vi "Multi_Point_TraverseControl.vi"(0 "Mode":T2=enum."Read traverse position", 1 "Route Checking?":bool, 3 "Traverse Name":string, 5 "RollPitchYaw":dbl[](array[numeric]) caption="Model       Roll      Pitch       Yaw (deg)" format="%#.2f", 9 "Points to plot":dbl[][](array[numeric]) format="%.2f", 11 "Work in Tunnel Coordinates?":T1, 13 "Speed Factor":dbl=1.0 min=0.1 max=5.0 format="%.2f", 14 "Backlash Compensation?":bool=TRUE) -> (4 "Position Output XYZ":dbl[](array[numeric]) format="%.2f", 15 "Error String":string)   [LabVIEW 2013]
uses:
  Anemometry/Anemometry Sub Vis/Gen Trav/Trav_mode.ctl
  Anemometry/Anemometry Sub Vis/Controls/Tunnel_Coordinates.ctl
  ~subVIs/GenericDriveCommand.ctl
  ADAM Client/Sub VIs/ADAM Controls/Update_scan_value.ctl
  Anemometry/Anemometry Sub Vis/Globals/Trav_pos_global.vi
  Anemometry/Anemometry Sub Vis/Globals/Preference_global.vi
  ~subVIs/DriveConfigGlobal.vi
  Anemometry/Anemometry Sub Vis/Gen Trav/Route mapping/Route_mapping_global.vi
panel:
  out "Server copy Location":path
  out "Log File":path
  out "Achieved Pos In Eng units of all channels":dbl[](array[numeric]) format="%.2f"
  out "Pulses Positon all channels":dbl[](array[numeric])
  out "Counters Reset?":bool
  # "X                Y                   Z"
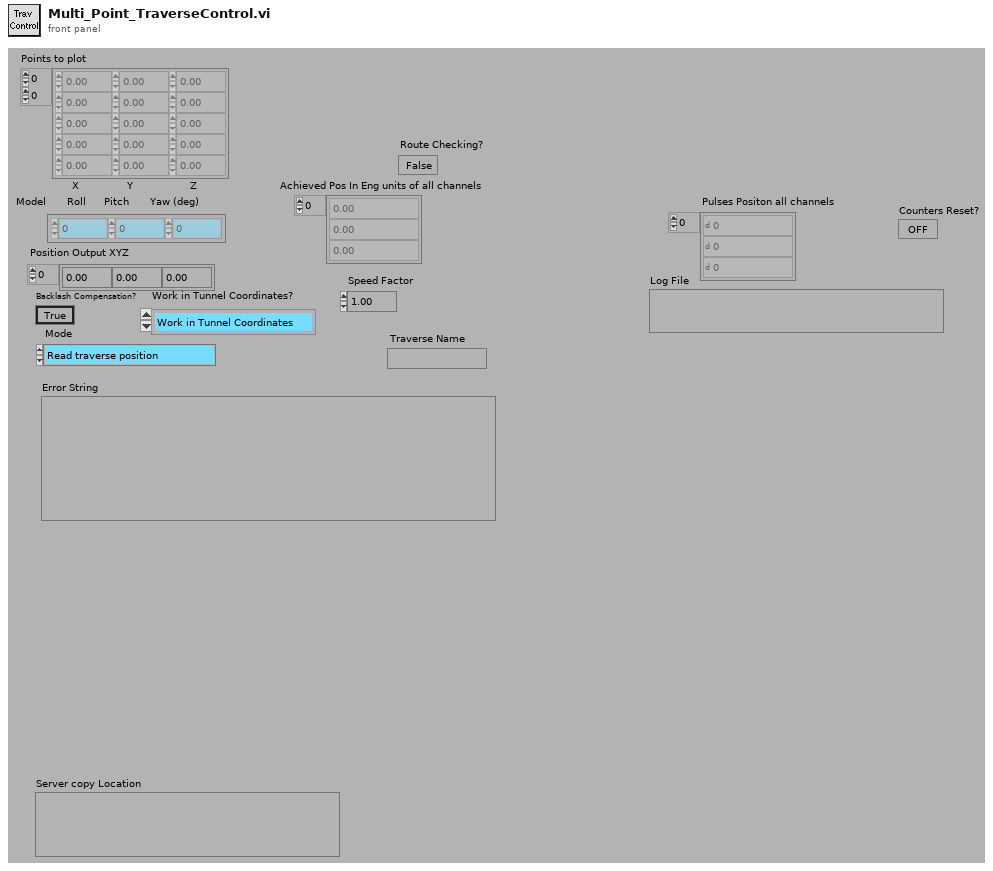
[diagram p1: front panel]
types:
  T1 = typedef "Tunnel_Coordinates.ctl" = enum16{"Work in Tunnel Coordinates", "Work in Model Coordinates"}
  T2 = typedef "Trav_mode.ctl" = enum16{"Move traverse", "Read traverse position", "Teach Position"}
  T3 = typedef "GenericDriveCommand.ctl" = string
  T4 = enum16{"To Traverse Coordinates", "To User Coordinates"}
  T5 = typedef "Update_scan_value.ctl" = cluster{"Channel Name":string, "New Value":dbl}
  T6 = typedef "AxisConfigCluster.ctl" = cluster{"Channel Properties":T7, "Static Drive Configuration":T8}
  T7 = typedef "DriveProperties.ctl" = cluster{"Channel Name":string, "Vel. Default":dbl, "Acc. Default":dbl, "Vel. Max":dbl, "Vel. Min":dbl, "Acc. Max":dbl, "Acc. Min":dbl, "Pulses/unit":dbl, "Address":u8, "Pulse Offset":i32, "Pos Tolerance":dbl, "Pulses/rev":dbl, "Backlash/Eng units":dbl, "Current Pos":dbl, "Ch Status":enum16{"Active", "Offline", "Simulate"}, "Port Name":string, "Axis Transform mode":string, "Metadata Ch Name":string, "Type":string}
  T8 = typedef "DriveStaticConfig.ctl" = cluster{"Correction Gain % (CG)":u16, "Dead Band (DB)":i32, "Dead Band Window (DW)":i32, "Encoder Resolution (ER)":i32, "Step Mode  (FSB)":u16, "Position Maintenance (FSC)":u16, "Stop on Stall (FSD)":u16, "Activate OP1 on stall (FSE)":u16, "Stop on Trigger 3 (FSF)":u16, "OP2 in Deadband (FSG)":u16, "Stall Detect (FSH)":u16, "Limit Disable (LD)":u16, "Motor Resolution (MR)":enum16{"200", "400", "1000", "2000", "4000", "5000", "10000", "12800", "18000", "20000", "21600", "25000", "25400", "25600", "36000", "50000", "278528", "425984", "507904", "614400", "655360", "819200", "1024000"}, "Limit Switch Sense (OSA)":u16, "Home Position (OSB)":u16, "Home Switch Sense (OSC)":u16, "Encoder Z for Home (OSD)":u16, "Reference edge of Home (OSH)":u16, "RS232 Echo Control (SSA)":u16, "Buffer at Limit (SSG)":u16, "Buffer at Stop (SSH)":u16, "Indexer Mode  (FSA)":u16, "Type":string, "ConfigString":string, "De Power Motor":enum16{"TRUE", "FALSE"}}
  T9 = typedef "Box_size.ctl" = cluster{"Max":dbl, "Min":dbl}[]
  T10 = typedef "Exclude_cluster.ctl" = cluster{"Sizes":T9, "Name":string, "Exclude Type":T11}
  T11 = typedef "Exclusion_type.ctl" = enum16{"Exclude completely", "Allow only vertical moves"}
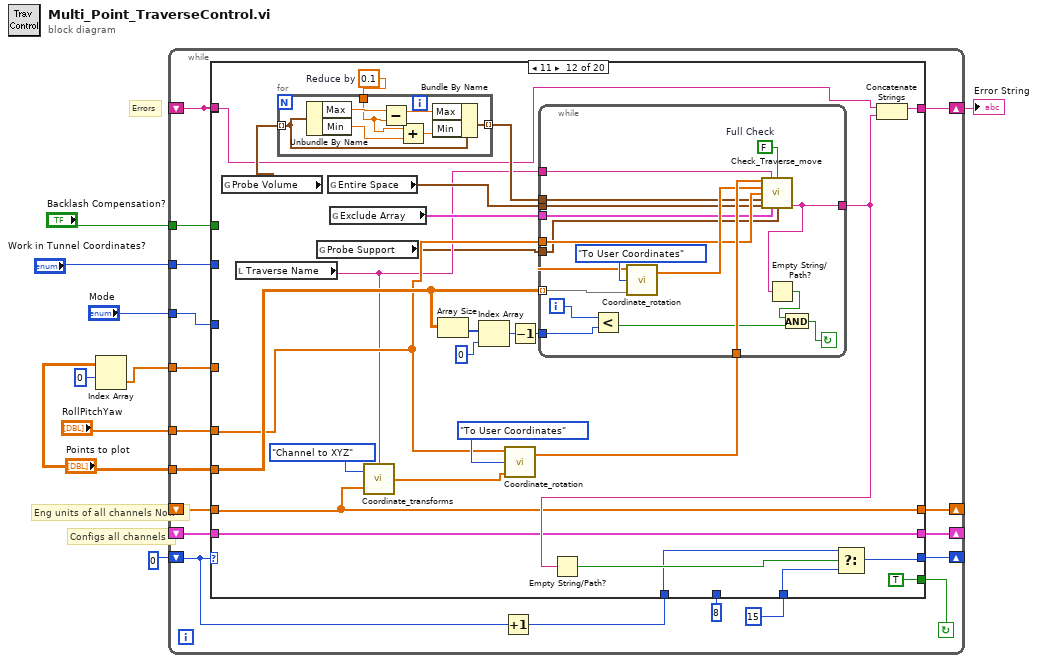
[diagram p0: block diagram]
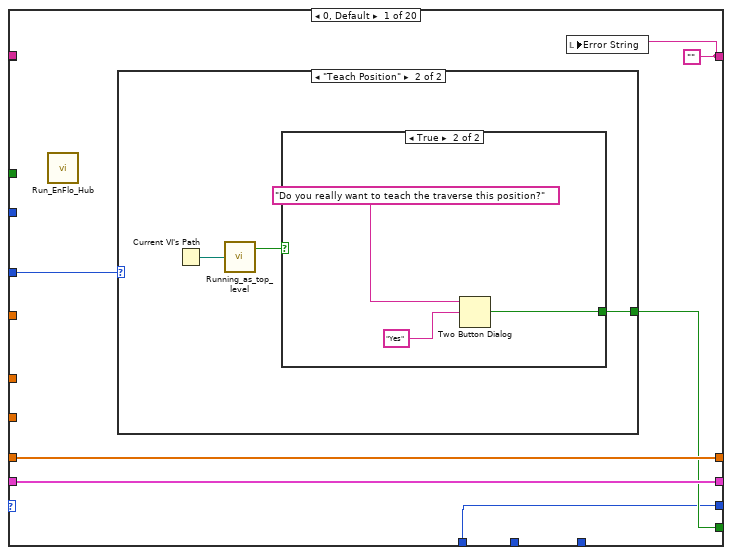
[diagram p2: hidden frame]
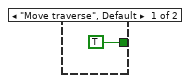
[diagram p3: hidden frame]
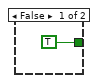
[diagram p4: hidden frame]
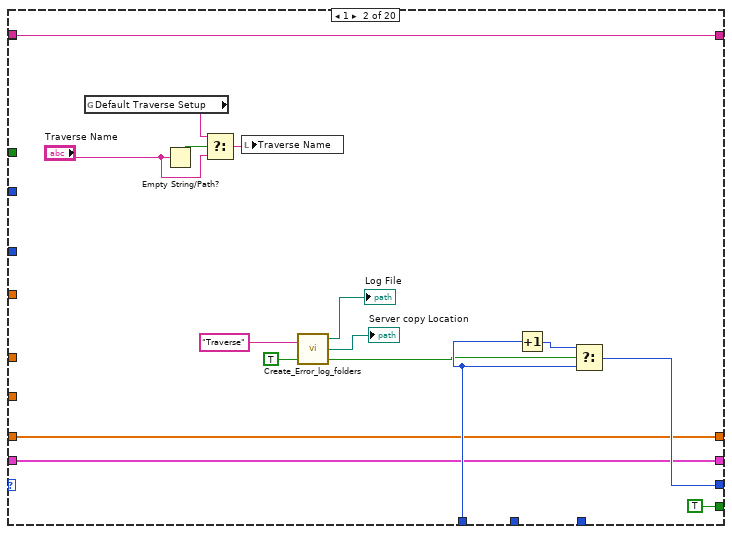
[diagram p5: hidden frame]
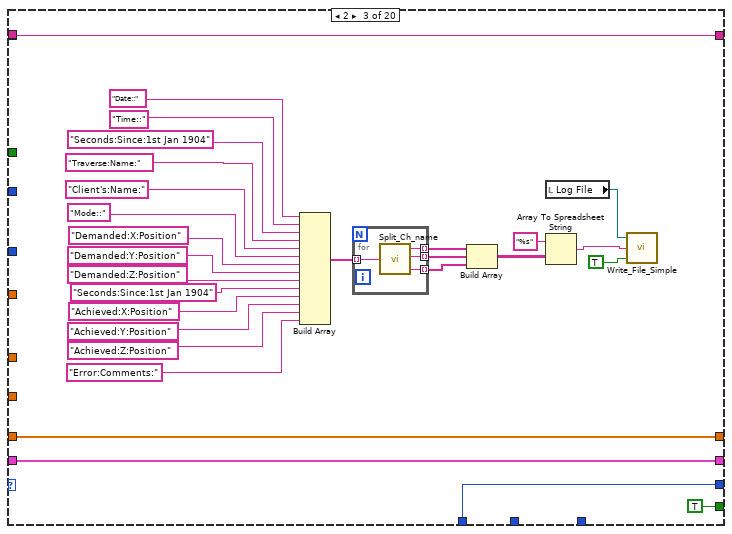
[diagram p6: hidden frame]
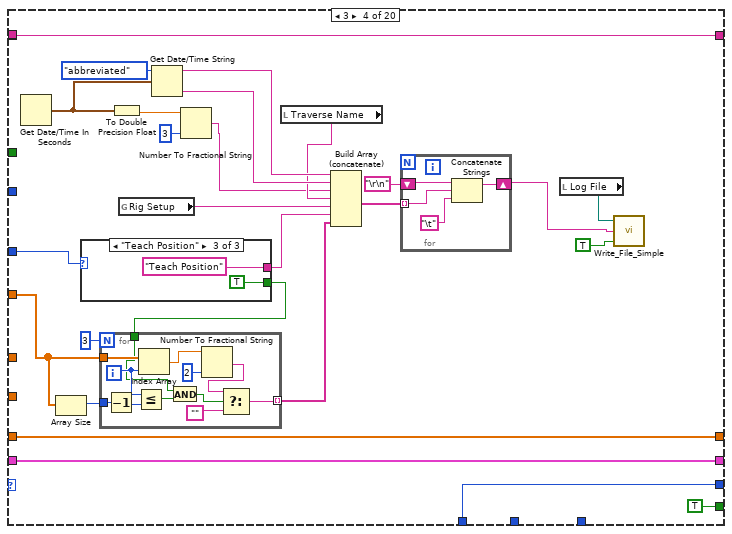
[diagram p7: hidden frame]
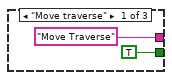
[diagram p8: hidden frame]
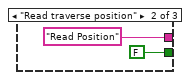
[diagram p9: hidden frame]
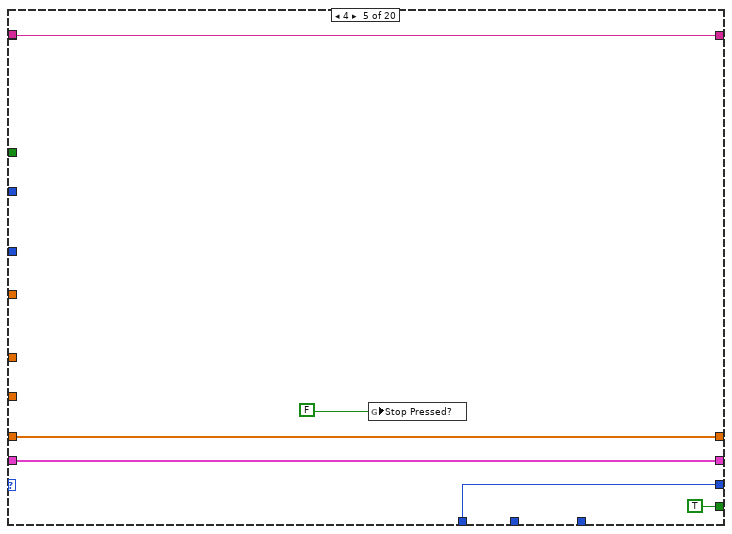
[diagram p10: hidden frame]
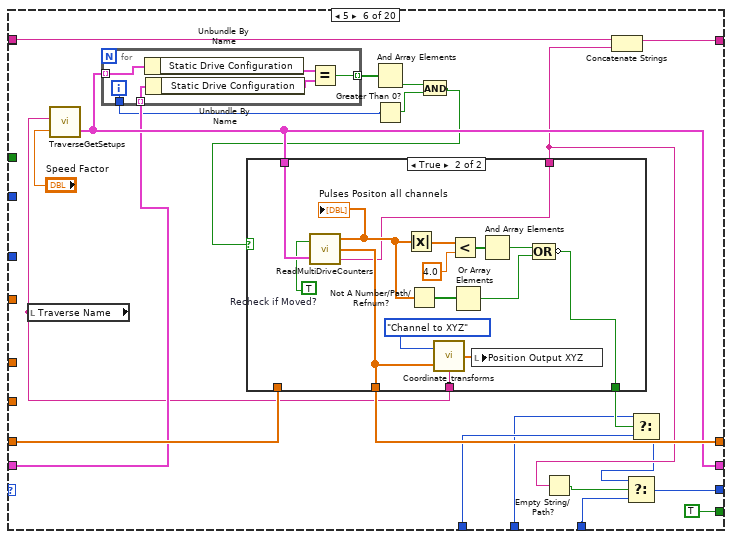
[diagram p11: hidden frame]
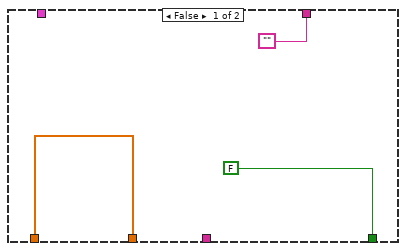
[diagram p12: hidden frame]
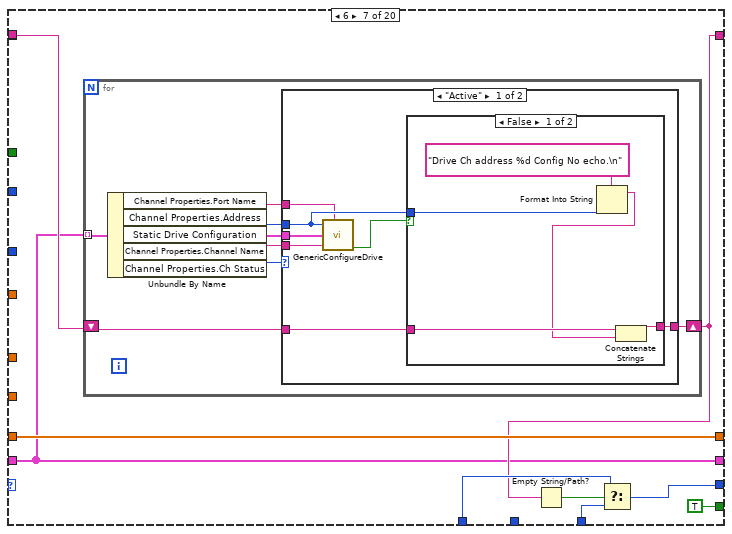
[diagram p13: hidden frame]
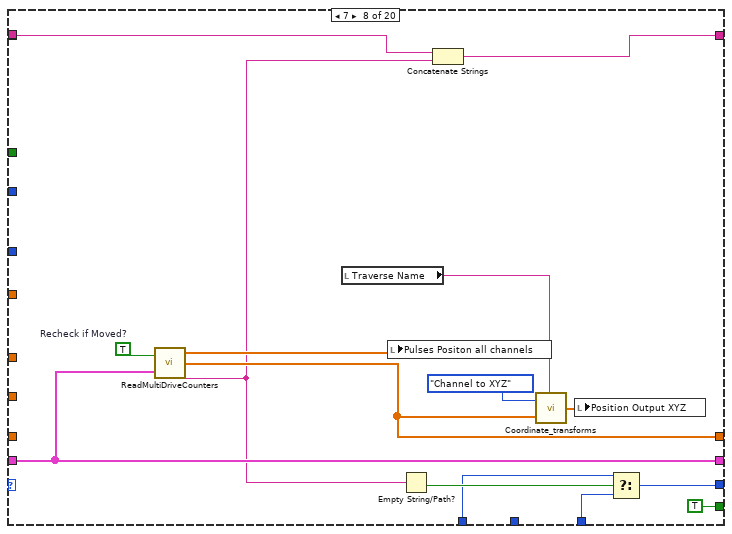
[diagram p16: hidden frame]
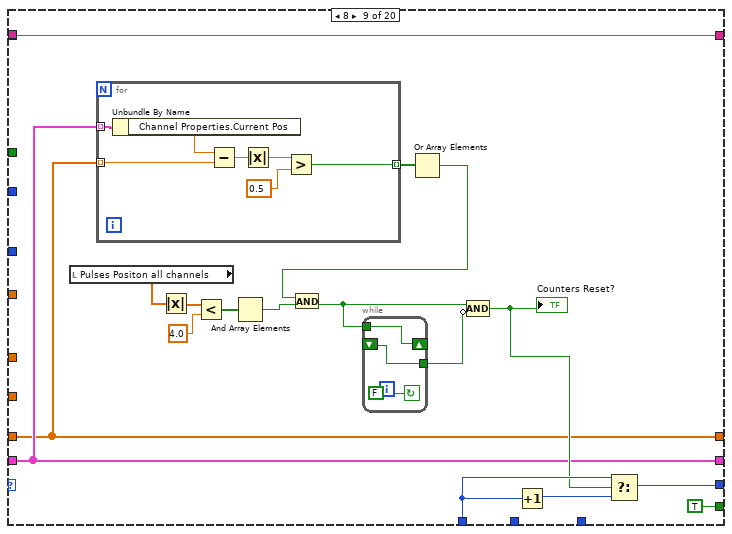
[diagram p17: hidden frame]
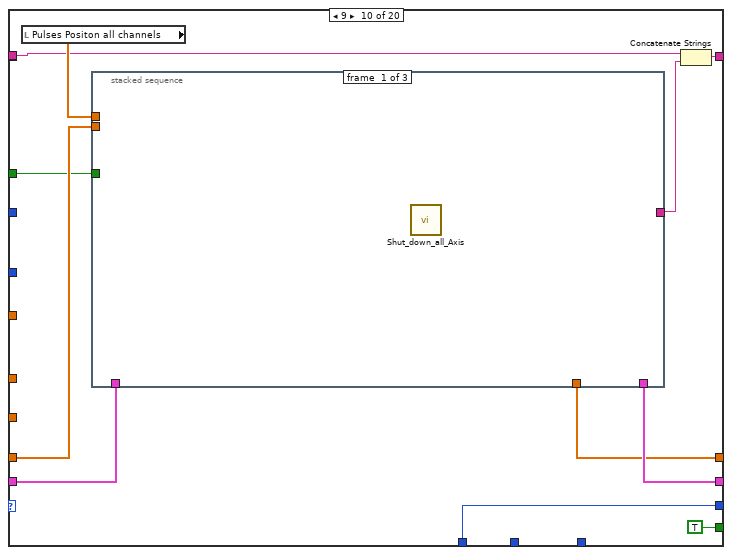
[diagram p18: hidden frame]
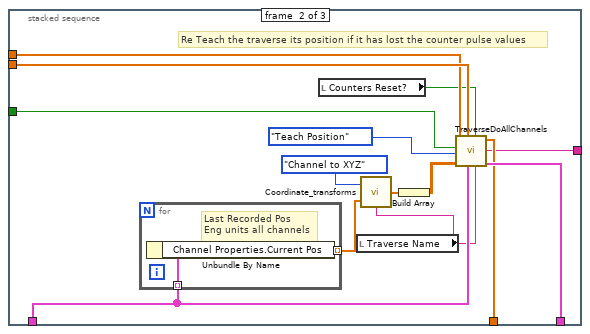
[diagram p19: hidden frame]
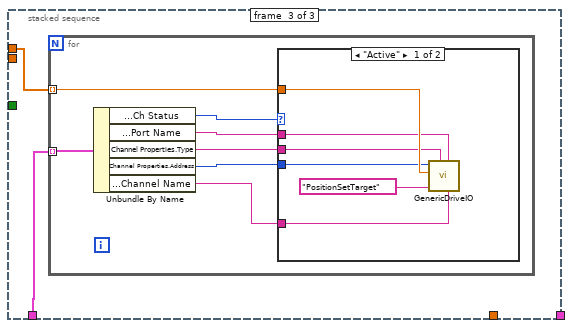
[diagram p20: hidden frame]
diagram:
  # "Errors"
  # "Eng units of all channels Now"
  # "Configs all channels"
  n1 = Index Array(array="Points to plot", index (row)=0) -> (element=w4:dbl[])  [unwired: 1 in]
  n2 = while {
    tunnel: "Backlash Compensation?" -> [w13]
    tunnel: w4 -> [w17]
    shift-left: _ -> [w14]
    shift-right: [w18] -> w7
    shift-left: _ -> [w19]
    shift-right: [w20] -> _
    shift-left: _ -> [w21]
    shift-right: [w22] -> _
    shift-left: 0 -> [w25]
    shift-right: [w23] -> _
    tunnel: "Mode" -> [w27]
    tunnel: "RollPitchYaw" -> [w12]
    tunnel: "Work in Tunnel Coordinates?" -> [w11]
    tunnel: "Points to plot" -> [w10]
    stop <- w26 continue-if-true
    n3 = Increment(x=w25) -> (x+1=w24:i32)
    n4 = case shown="11" w25 {
      tunnel: w27 -> [w33 _ _ w108 _ _ _ _ _ _ w310 _ w375 w405 _ _ _ w481 _ w537]
      tunnel: [w30 TRUE ("T button?") TRUE ("T button?") TRUE ("T button?") TRUE TRUE ("T button?") TRUE ("T button?") TRUE ("T button?") TRUE TRUE TRUE ("T button?") TRUE ("T button?") TRUE TRUE TRUE ("T button?") TRUE ("T button?") TRUE ("T button?") w483 TRUE FALSE] -> w26
      tunnel: w24 -> [w29 w56 w65 w113 w138 w162 w195 w223 w248 w264 w309 w325 w382 w407 w433 w447 w476 w480 w515 w544]
      tunnel: [w29 w54 w65 w113 w138 w145 w194 w221 w246 w264 w308 w323 w382 w406 w433 w445 w476 w479 w515 w544] -> w23
      tunnel: [w31 w51 w67 w115 w140 w160 w190 w235 w242 w273 w306 w329 w376 w404 w435 w459 w478 w486 w513 w542] -> w22
      tunnel: w21 -> [w31 w51 w67 w115 w140 w159 w190 w235 w242 w272 w306 w329 w389 w404 w435 w459 w478 w486 w513 w542]
      tunnel: [w32 w52 w66 w114 w141 w165 w198 w230 w241 w269 w305 w328 w383 w410 w434 w458 w477 w487 w516 w545] -> w20
      tunnel: w19 -> [w32 w52 w66 w114 w141 w164 w198 _ w241 w270 w305 w328 w378 w410 w434 w458 w477 w487 w516 w545]
      tunnel: [w28 w50 w63 w105 w142 w150 w191 w226 w245 w266 w311 w326 w385 w408 w431 w449 w474 w482 w509 w538] -> w18
      tunnel: w14 -> [_ w50 w63 w105 w142 w151 w192 w227 w245 w268 w311 w327 w386 w408 w431 w449 w474 w485 w511 w540]
      tunnel: w17 -> [_ _ _ w102 _ _ _ _ _ _ _ _ _ _ _ _ _ _ w507 _]
      tunnel: 15 ("f") -> [_ _ _ _ _ w146 w193 w222 _ _ _ w324 _ _ _ _ _ _ _ _]
      tunnel: 8 ("t") -> [_ _ _ _ _ w161 _ _ _ _ _ _ _ _ _ _ _ _ _ _]
      tunnel: w14 -> [_ _ _ _ _ _ _ _ _ _ _ _ _ _ _ _ _ _ _ _]
      tunnel: w13 -> [_ _ _ _ _ _ _ _ _ w263 _ _ w377 _ _ _ _ _ _ _]
      tunnel: w12 -> [_ _ _ _ _ _ _ _ _ _ _ w330 w373 _ _ _ _ _ w508 w535]
      tunnel: w11 -> [_ _ _ _ _ _ _ _ _ _ _ _ w372 _ _ _ _ _ w505 w533]
      tunnel: w10 -> [_ _ _ _ _ _ _ _ _ _ _ w331 w374 _ _ _ _ _ _ _]
      frame 0, Default {
        w28 = ""
        n5 = call "Run_EnFlo_Hub.vi"() -> ()  [unwired: 8 out]
        n6 = case shown="\"Teach Position\"" w33 {
          tunnel: [TRUE ("T button?") w35] -> w30
          frame "Move traverse", Default {
          }
          frame "Teach Position" {
            n7 = Current VI's Path() -> (path=w37:path)
            n8 = call "Running_as_top_level.vi"("Vi path name"=w37) -> ("Top Level"=w36:bool)  [unwired: 1 out]
            n9 = case shown="True" w36 {
              tunnel: [TRUE ("T button?") w39] -> w35
              frame False {
              }
              frame True {
                n10 = Two Button Dialog(message="Do you really want to teach the traverse this position?", 2:"Yes" ("T button name (\"OK\")")) -> (T button?=w39:bool)  [unwired: 1 out]
              }
            }
          }
        }
        n11 = local write "Error String"(w28) -> ()
      }
      frame 1 {
        n12 = global read "Trav_pos_global.vi" "Default Traverse Setup"() -> (w47:string)
        n13 = Empty String/Path?(string/path="Traverse Name") -> (empty?=w45:bool)
        n14 = Select(t=w47, s=w45, f="Traverse Name") -> (s? t:f=w44:string)
        n15 = local write "Traverse Name"(w44) -> ()
        n16 = call "Create_Error_log_folders.vi"("Per Day Log File?"=TRUE, "Log Filename"="Traverse" ("Input Element")) -> ("exists?"=w48:bool, "Server copy Location"=→"Server copy Location":path, "Local Log File"=→"Log File":path)  [unwired: 1 in]
        n17 = Increment(x=w56) -> (x+1=w55:i32)
        n18 = Select(t=w55, s=w48, f=w56) -> (s? t:f=w54:i32)
      }
      frame 2 {
        n19 = Build Array("Date::", "Time::", "Seconds:Since:1st Jan 1904", "Traverse:Name:", "Client's:Name:", "Mode::", "Demanded:X:Position", "Demanded:Y:Position", "Demanded:Z:Position", "Seconds:Since:1st Jan 1904", "Achieved:X:Position", "Achieved:Y:Position", "Achieved:Z:Position", "Error:Comments:") -> (w70:string[])
        n20 = for {
          tunnel: w70 -> [w89] mode=indexing
          tunnel: [w88] -> w71 mode=indexing
          tunnel: [w87] -> w72 mode=indexing
          tunnel: [w86] -> w73 mode=indexing
          n21 = call "Split_Ch_name.vi"("Ch name"=w89) -> ("Top level"=w88:string, "Middle"=w87:string, "Low level"=w86:string)
        }
        n22 = Build Array(w71, w72, w73) -> (w68:string[][])
        n23 = local read "Log File"() -> (w59:path)
        n24 = Array To Spreadsheet String(array=w68, 3:"%s" ("format string")) -> (spreadsheet string=w60:string)  [unwired: 1 out]
        n25 = call "Write_File_Simple.vi"("append to file? (new file:F)"=TRUE, "character string"=w60, "file path"=w59) -> ()  [unwired: 2 out]
      }
      frame 3 {
        n26 = Get Date/Time In Seconds() -> (seconds since 1Jan1904=w94:timestamp)
        n27 = Array Size(array=w102) -> (size(s)=w103:i32)
        n28 = case shown="\"Teach Position\"" w108 {
          tunnel: ["Move Traverse" "Read Position" "Teach Position"] -> w109
          tunnel: [TRUE FALSE TRUE] -> w99
          frame "Move traverse" {
          }
          frame "Read traverse position" {
          }
          frame "Teach Position" {
          }
        }
        n29 = for {
          N: 3 -> [_]
          tunnel: w102 -> [w127]
          tunnel: w103 -> [w124]
          tunnel: [w120] -> w100 mode=indexing
          tunnel: w99 -> [w116]
          i -> [w122]
          n30 = Decrement(x=w124) -> (x-1=w123:i32)
          n31 = Less Or Equal?(x=w122, y=w123) -> (x <= y?=w118:bool)
          n32 = Index Array(array=w127, index=w122) -> (element=w126:dbl)
          n33 = And(x=w116, y=w118) -> (x .and. y?=w117:bool)
          n34 = Number To Fractional String(number=w126, precision (6)=i16 2) -> (F-format string=w121:string)  [unwired: 2 out]
          n35 = Select(t=w121, s=w117, f="") -> (s? t:f=w120:string)
        }
        n36 = To Double Precision Float(number=w94) -> (double precision float=w93:dbl)
        n37 = global read "Preference_global.vi" "Rig Setup"() -> (w90:string)
        n38 = Get Date/Time String(date format (0)=enum16{"short", "long", "abbreviated"}."abbreviated", seconds (now)=w94) -> (date string=w111:string, time string=w110:string)  [unwired: 1 out]
        n39 = Number To Fractional String(number=w93, precision (6)=i16 3) -> (F-format string=w91:string)  [unwired: 2 out]
        n40 = local read "Traverse Name"() -> (w95:string)
        n41 = Build Array (concatenate)(w111, w110, w91, w95, w90, w109, w100) -> (w106:string[])
        n42 = for {
          shift-right: [w130] -> w96
          shift-left: "\r\n" -> [w131]
          tunnel: w106 -> [w129] mode=indexing
          n43 = Concatenate Strings(w131, w129, "\t") -> (w130:string)
        }
        n44 = local read "Log File"() -> (w97:path)
        n45 = call "Write_File_Simple.vi"("append to file? (new file:F)"=TRUE, "character string"=w96, "file path"=w97) -> ()  [unwired: 2 out]
      }
      frame 4 {
        n46 = global write "DriveConfigGlobal.vi" "Stop Pressed?"(FALSE) -> ()
      }
      frame 5 {
        n47 = local read "Traverse Name"() -> (w153:string)
        n48 = call "TraverseGetSetups.vi"("Speed Factor"="Speed Factor", "Traverse Name"=w153) -> ("Matched Configurations"=w160:T6[])  [unwired: 1 out]
        n49 = for {
          tunnel: w160 -> [w171] mode=indexing
          tunnel: w159 -> [w170] mode=indexing
          tunnel: [w167] -> w158 mode=indexing
          tunnel: [w166] -> w157
          i -> [w166]
          n50 = Unbundle By Name(w171) -> ("Static Drive Configuration"=w169:T8)
          n51 = Unbundle By Name(w170) -> ("Static Drive Configuration"=w168:T8)
          n52 = Equal?(x=w169, y=w168) -> (x = y?=w167:bool)
        }
        n53 = And Array Elements(Boolean array=w158) -> (logical AND=w155:bool)
        n54 = Greater Than 0?(x=w157) -> (x > 0?=w156:bool)
        n55 = And(x=w155, y=w156) -> (x .and. y?=w154:bool)
        n56 = case shown="True" w154 {
          tunnel: w160 -> [_ w189]
          tunnel: [w174 w179] -> w165
          tunnel: w164 -> [w174 _]
          tunnel: [FALSE w181] -> w163
          tunnel: w153 -> [_ w177]
          tunnel: ["" w175] -> w149
          frame False {
          }
          frame True {
            w176 = TRUE  # Recheck if Moved?
            n57 = call "ReadMultiDriveCounters.vi"("Recheck if Moved?"=w176, "Matched Configurations"=w189) -> ("Pulses"=w184:dbl[], "Eng units"=w179:dbl[], "Error String"=w175:string)
            "Pulses Positon all channels" <- w184
            n58 = Absolute Value(x=w184) -> (abs(x)=w188:dbl[])
            n59 = Not A Number/Path/Refnum?(number/path/refnum=w184) -> (NaN/Path/Refnum?=w183:bool[])
            n60 = call "Coordinate_transforms.vi"("Traverse Name"=w177, "Input"=w179, "Mode"=enum16{"XYZ to Channel", "Channel to XYZ"}."Channel to XYZ") -> ("Output"=w178:dbl[])
            n61 = Less?(x=w188, y=4.0 ("Achieved Position")) -> (x < y?=w186:bool[])
            n62 = Or Array Elements(Boolean array=w183) -> (logical OR=w182:bool)
            n63 = local write "Position Output XYZ"(w178) -> ()
            n64 = And Array Elements(Boolean array=w186) -> (logical AND=w185:bool)
            n65 = Compound Arithmetic op=OR(w185, w182) -> (invert w181:bool)
          }
        }
        n66 = Empty String/Path?(string/path=w149) -> (empty?=w148:bool)
        n67 = Concatenate Strings(w151, w149) -> (w150:string)
        n68 = Select(t=w161, s=w163, f=w162) -> (s? t:f=w147:i32)
        n69 = Select(t=w147, s=w148, f=w146) -> (s? t:f=w145:i32)
      }
      frame 6 {
        n70 = for {
          tunnel: w190 -> [w206] mode=indexing
          shift-right: [w199] -> w191
          shift-left: w192 -> [w200]
          n71 = Unbundle By Name(w206) -> ("Channel Properties.Port Name"=w201:string, "Channel Properties.Address"=w205:u8, "Static Drive Configuration"=w204:T8, "Channel Properties.Channel Name"=w203:string, "Channel Properties.Ch Status"=w202:enum16{"Active", "Offline", "Simulate"})
          n72 = case shown="\"Active\"" w202 {
            tunnel: w205 -> [w211 _]
            tunnel: w204 -> [w213 _]
            tunnel: w203 -> [w212 _]
            tunnel: w201 -> [w210 _]
            tunnel: w200 -> [w208 w220]
            tunnel: [w207 w220] -> w199
            frame "Active" {
              n73 = call "GenericConfigureDrive.vi"("Address"=w211, "Port Name"=w210, "Static Drive Configuration"=w213, "Channel Name"=w212) -> ("Good Echo"=w209:bool)  [unwired: 4 out]
              n74 = case shown="False" w209 {
                tunnel: w211 -> [w218 _]
                tunnel: w208 -> [w216 w219]
                tunnel: [w215 w219] -> w207
                frame False {
                  n75 = Format Into String(format string="Drive Ch address %d Config No echo.\n" ("Format String"), w218) -> (resulting string=w214:string)  [unwired: 2 in, 1 out]
                  n76 = Concatenate Strings(w216, w214) -> (w215:string)
                }
                frame True {
                }
              }
            }
            frame "Offline", Default {
            }
          }
        }
        n77 = Empty String/Path?(string/path=w191) -> (empty?=w196:bool)
        n78 = Select(t=w195, s=w196, f=w193) -> (s? t:f=w194:i32)
      }
      frame 7 {
        w228 = TRUE  # Recheck if Moved?
        n79 = call "ReadMultiDriveCounters.vi"("Recheck if Moved?"=w228, "Matched Configurations"=w235) -> ("Pulses"=w233:dbl[], "Eng units"=w230:dbl[], "Error String"=w224:string)
        n80 = local read "Traverse Name"() -> (w229:string)
        n81 = local write "Pulses Positon all channels"(w233) -> ()
        n82 = Empty String/Path?(string/path=w224) -> (empty?=w225:bool)
        n83 = Concatenate Strings(w227, w224) -> (w226:string)
        n84 = call "Coordinate_transforms.vi"("Traverse Name"=w229, "Input"=w230, "Mode"=enum16{"XYZ to Channel", "Channel to XYZ"}."Channel to XYZ") -> ("Output"=w231:dbl[])
        n85 = local write "Position Output XYZ"(w231) -> ()
        n86 = Select(t=w223, s=w225, f=w222) -> (s? t:f=w221:i32)
      }
      frame 8 {
        n87 = local read "Pulses Positon all channels"() -> (w236:dbl[])
        n88 = for {
          tunnel: w242 -> [w262] mode=indexing
          tunnel: w241 -> [w260] mode=indexing
          tunnel: [w256] -> w239 mode=indexing
          n89 = Unbundle By Name(w262) -> ("Channel Properties.Current Pos"=w261:dbl)
          n90 = Subtract(x=w261, y=w260) -> (x-y=w259:dbl)
          n91 = Absolute Value(x=w259) -> (abs(x)=w258:dbl)
          n92 = Greater?(x=w258, y=0.5) -> (0:w256:bool)
        }
        n93 = Absolute Value(x=w236) -> (abs(x)=w252:dbl[])
        n94 = Less?(x=w252, y=4.0 ("Achieved Position")) -> (x < y?=w250:bool[])
        n95 = And Array Elements(Boolean array=w250) -> (logical AND=w240:bool)
        n96 = Or Array Elements(Boolean array=w239) -> (logical OR=w238:bool)
        n97 = And(x=w238, y=w240) -> (x .and. y?=w237:bool)
        n98 = while {
          tunnel: [w254] -> w244
          tunnel: w237 -> [w255]
          shift-left: _ -> [w254]
          shift-right: [w255] -> _
          stop <- FALSE continue-if-true
        }
        n99 = Compound Arithmetic op=AND(w237, invert w244) -> (w243:bool)
        "Counters Reset?" <- w243
        n100 = Increment(x=w248) -> (x+1=w247:i32)
        n101 = Select(t=w248, s=w243, f=w247) -> (s? t:f=w246:i32)
      }
      frame 9 {
        n102 = local read "Pulses Positon all channels"() -> (w271:dbl[])
        n103 = stacked-sequence {
          tunnel: w271 -> [_ w279 w290]
          tunnel: [_ w287 _] -> w273
          tunnel: w270 -> [_ w286 _]
          tunnel: [_ w285 _] -> w269
          tunnel: w272 -> [_ w281 w291]
          tunnel: [_ w284 _] -> w267
          tunnel: w263 -> [_ w275 _]
          frame #0 {
            n104 = call "Shut_down_all_Axis.vi"() -> ()  [unwired: 1 out]
          }
          frame #1 {
            # "Re Teach the traverse its position if it has lost the counter pulse values"
            n105 = for {
              tunnel: [w289] -> w280 mode=indexing
              tunnel: w281 -> [w288] mode=indexing
              # "Last Recorded Pos\nEng units all channels"
              n106 = Unbundle By Name(w288) -> ("Channel Properties.Current Pos"=w289:dbl)
            }
            n107 = local read "Counters Reset?"() -> (w277:bool)
            n108 = local read "Traverse Name"() -> (w276:string)
            n109 = call "Coordinate_transforms.vi"("Traverse Name"=w276, "Input"=w280, "Mode"=enum16{"XYZ to Channel", "Channel to XYZ"}."Channel to XYZ") -> ("Output"=w282:dbl[])
            n110 = Build Array(w282) -> (w274:dbl[][])
            n111 = call "TraverseDoAllChannels.vi"("Traverse Name"=w276, "Counters Reset?"=w277, "Matched Configurations all Channels In"=w281, "Current Pos In Eng units of all channels"=w286, "Position Steps"=w274, "Mode"=Trav_mode."Teach Position", "Backlash Compensation?"=w275, "Current Pulses positions for all channels"=w279) -> ("Matched Configurations Out"=w287:T6[], "Error String"=w284:string, "Achieved Pos In Eng units of all channels"=w285:dbl[])  [unwired: 1 out]
          }
          frame #2 {
            n112 = for {
              tunnel: w291 -> [w298] mode=indexing
              tunnel: w290 -> [w297] mode=indexing
              n113 = Unbundle By Name(w298) -> ("Channel Properties.Ch Status"=w296:enum16{"Active", "Offline", "Simulate"}, "Channel Properties.Port Name"=w295:string, "Channel Properties.Type"=w294:string, "Channel Properties.Address"=w293:u8, "Channel Properties.Channel Name"=w292:string)
              n114 = case shown="\"Active\"" w296 {
                tunnel: w297 -> [w304 _]
                tunnel: w295 -> [w303 _]
                tunnel: w294 -> [w302 _]
                tunnel: w293 -> [w301 _]
                tunnel: w292 -> [w300 _]
                frame "Active" {
                  n115 = call "GenericDriveIO.vi"("GenericDriveCommand"=T3 "PositionSetTarget", "Channel Name"=w300, "Numeric Value"=w304, "Address"=w301, "Type"=w302, "Port Name"=w303) -> ()  [unwired: 1 in, 5 out]
                }
                frame "Offline", Default {
                }
              }
            }
          }
        }
        n116 = Concatenate Strings(w268, w267) -> (w266:string)
      }
      frame 10 {
        n117 = case shown="\"Move traverse\"" w310 {
          tunnel: w309 -> [w312 w319]
          tunnel: [w314 w318] -> w308
          frame "Move traverse" {
            n118 = Increment(x=w312) -> (x+1=w313:i32)
            n119 = case shown="True" "Route Checking?" {
              tunnel: [w316 w317] -> w314
              tunnel: w313 -> [w316 _]
              tunnel: w312 -> [_ w317]
              frame False {
              }
              frame True {
              }
            }
          }
          frame "Read traverse position", Default {
            n120 = Increment(x=w319) -> (x+1=w318:i32)
          }
        }
      }
      frame 11 {
        w340 = 0.1  # Reduce by
        n121 = global read "Route_mapping_global.vi" "Probe Volume"() -> (w341:T9)
        n122 = local read "Traverse Name"() -> (w322:string)
        n123 = for {
          tunnel: w341 -> [w370] mode=indexing
          tunnel: [w369] -> w342 mode=indexing
          tunnel: w340 -> [w364]
          n124 = Unbundle By Name(w370) -> ("Max"=w368:dbl, "Min"=w366:dbl)
          n125 = Subtract(x=w368, y=w364) -> (x-y=w367:dbl)
          n126 = Add(x=w364, y=w366) -> (x+y=w365:dbl)
          n127 = Bundle By Name(cluster=w370, "Max"=w367, "Min"=w365) -> (w369:cluster{"Max":dbl, "Min":dbl})
        }
        n128 = global read "Route_mapping_global.vi" "Probe Support"() -> (w320:T9)
        n129 = global read "Route_mapping_global.vi" "Entire Space"() -> (w339:T9)
        n130 = global read "Route_mapping_global.vi" "Exclude Array"() -> (w338:T10[])
        n131 = call "Coordinate_transforms.vi"("Traverse Name"=w322, "Input"=w328, "Mode"=enum16{"XYZ to Channel", "Channel to XYZ"}."Channel to XYZ") -> ("Output"=w336:dbl[])
        n132 = Array Size(array=w331) -> (size(s)=w343:i32[])
        n133 = Index Array(array=w343, index=0) -> (element=w345:i32)
        n134 = call "Coordinate_rotation.vi"("Model       Roll      Pitch       Yaw (deg)"=w330, "Input Position"=w336, "Mode"=T4."To User Coordinates") -> ("Output Position"=w333:dbl[])  [unwired: 2 in, 1 out]
        n135 = Decrement(x=w345) -> (x-1=w346:i32)
        n136 = while {
          tunnel: w333 -> [w362]
          tunnel: w331 -> [w360] mode=indexing
          tunnel: w322 -> [w359]
          tunnel: w330 -> [w357]
          tunnel: [w353] -> w337
          tunnel: w338 -> [w356]
          tunnel: w339 -> [w355]
          tunnel: w342 -> [w354]
          tunnel: w346 -> [w351]
          tunnel: w320 -> [w347]
          i -> [w352]
          stop <- w348 continue-if-true
          w358 = FALSE  # Full Check
          n137 = Less?(x=w352, y=w351) -> (x < y?=w349:bool)
          n138 = call "Coordinate_rotation.vi"("Model       Roll      Pitch       Yaw (deg)"=w357, "Input Position"=w360, "Mode"=T4."To User Coordinates") -> ("Output Position"=w361:dbl[])  [unwired: 2 in, 1 out]
          n139 = call "Check_Traverse_move.vi"("Current position"=w362, "Traverse Name"=w359, "Full Check"=w358, "New Position"=w361, "Model       Roll      Pitch       Yaw (deg)"=w357, "Probe Volume"=w354, "Entire Space"=w355, "Exclude Array"=w356, "Probe Support"=w347) -> ("Error Comments"=w353:string)  [unwired: 6 out]
          n140 = Empty String/Path?(string/path=w353) -> (empty?=w350:bool)
          n141 = And(x=w350, y=w349) -> (x .and. y?=w348:bool)
        }
        n142 = Empty String/Path?(string/path=w337) -> (empty?=w334:bool)
        n143 = Select(t=w325, s=w334, f=w324) -> (s? t:f=w323:i32)
        n144 = Concatenate Strings(w327, w337) -> (w326:string)
      }
      frame 12 {
        w380 = FALSE  # Counters Reset?
        n145 = case shown="\"Work in Model Coordinates\"" w372 {
          tunnel: w373 -> [_ w394]
          tunnel: w374 -> [w391 w393]
          tunnel: [w391 w392] -> w371
          frame "Work in Tunnel Coordinates" {
          }
          frame "Work in Model Coordinates" {
            n146 = for {
              tunnel: w393 -> [w397] mode=indexing
              tunnel: [w396] -> w392 mode=indexing
              tunnel: w394 -> [w395]
              n147 = call "Coordinate_rotation.vi"("Model       Roll      Pitch       Yaw (deg)"=w395, "Input Position"=w397, "Mode"=T4."To Traverse Coordinates") -> ("Output Position"=w396:dbl[])  [unwired: 2 in, 1 out]
            }
          }
        }
        n148 = local read "Pulses Positon all channels"() -> (w390:dbl[])
        n149 = local read "Traverse Name"() -> (w379:string)
        n150 = call "TraverseDoAllChannels.vi"("Traverse Name"=w379, "Counters Reset?"=w380, "Matched Configurations all Channels In"=w389, "Current Pos In Eng units of all channels"=w378, "Position Steps"=w371, "Mode"=w375, "Backlash Compensation?"=w377, "Current Pulses positions for all channels"=w390) -> ("Matched Configurations Out"=w376:T6[], "Error String"=w384:string, "Achieved Pos In Eng units of all channels"=w383:dbl[])  [unwired: 1 out]
        "Achieved Pos In Eng units of all channels" <- w383
        n151 = call "Coordinate_transforms.vi"("Traverse Name"=w379, "Input"=w383, "Mode"=enum16{"XYZ to Channel", "Channel to XYZ"}."Channel to XYZ") -> ("Output"=→"Position Output XYZ":dbl[])
        n152 = Concatenate Strings(w386, w384) -> (w385:string)
      }
      frame 13 {
        n153 = local read "Position Output XYZ"() -> (w402:dbl[])
        n154 = case shown="\"Read traverse position\"" w405 {
          tunnel: w402 -> [_ _ _]
          frame "Move traverse" {
          }
          frame "Read traverse position" {
          }
          frame "Teach Position" {
            n155 = local write "Mode"(Trav_mode."Teach Position" ("Mode")) -> ()
          }
        }
        n156 = for {
          tunnel: w404 -> [w422] mode=indexing
          tunnel: T5 {"Channel Name"="", "New Value"=0.0} ("Update Scan Value Cluster") -> [w421]
          tunnel: w402 -> [w419] mode=indexing
          shift-right: [w417] -> w400
          shift-left: T5[] [] -> [w418]
          n157 = Unbundle By Name(w422) -> ("Channel Properties.Metadata Ch Name"=w420:string, "Channel Properties.Ch Status"=w416:enum16{"Active", "Offline", "Simulate"})
          n158 = Equal?(x=w416, y=enum16{"Active", "Offline", "Simulate"}."Active" ("Channel Properties.Ch Status")) -> (x = y?=w414:bool)
          n159 = Empty String/Path?(string/path=w420) -> (empty?=w413:bool)
          n160 = Compound Arithmetic op=AND(invert w413, w414) -> (w412:bool)
          n161 = case shown="True" w412 {
            tunnel: w421 -> [_ w429]
            tunnel: w420 -> [_ w428]
            tunnel: w419 -> [_ w427]
            tunnel: w418 -> [w423 w425]
            tunnel: [w423 w424] -> w417
            frame False {
            }
            frame True {
              n162 = Bundle By Name(cluster=w429, "Channel Name"=w428, "New Value"=w427) -> (w426:T5)
              n163 = Build Array (concatenate)(w425, w426) -> (w424:T5[])
            }
          }
        }
        n164 = global write "DriveConfigGlobal.vi" "Run Emergency stop loop"(FALSE ("Run Emergency stop loop")) -> ()
        n165 = Increment(x=w407) -> (x+1=w406:i32)
        n166 = call "Update_Current_Value_client.vi"("Don't Bother with check?"=FALSE, "Update array in"=w400) -> ()
      }
      frame 14 {
      }
      frame 15 {
        n167 = local read "Position Output XYZ"() -> (w453:dbl[])
        n168 = Array Size(array=w453) -> (size(s)=w452:i32)
        n169 = Get Date/Time In Seconds() -> (seconds since 1Jan1904=w444:timestamp)
        n170 = for {
          N: 3 -> [_]
          tunnel: w453 -> [w473]
          tunnel: w452 -> [w470]
          tunnel: [w465] -> w451 mode=indexing
          i -> [w468]
          n171 = Decrement(x=w470) -> (x-1=w469:i32)
          n172 = Less Or Equal?(x=w468, y=w469) -> (x <= y?=w467:bool)
          n173 = Index Array(array=w473, index=w468) -> (element=w472:dbl)
          n174 = Number To Fractional String(number=w472, precision (6)=i16 2) -> (F-format string=w466:string)  [unwired: 2 out]
          n175 = Select(t=w466, s=w467, f="") -> (s? t:f=w465:string)
        }
        n176 = To Double Precision Float(number=w444) -> (double precision float=w437:dbl)
        n177 = Number To Fractional String(number=w437, precision (6)=i16 3) -> (F-format string=w436:string)  [unwired: 2 out]
        n178 = call "Remove_unprintable_Char.vi"("Input String"=w449) -> ("Output String"=w450:string)
        n179 = Build Array (concatenate)(w436, w451, w450) -> (w455:string[])
        n180 = local read "Route Checking?"() -> (w448:bool)
        n181 = for {
          shift-right: [w462] -> w441
          shift-left: "" -> [w463]
          tunnel: w455 -> [w461] mode=indexing
          n182 = Concatenate Strings(w463, w461, "\t") -> (w462:string)
        }
        n183 = Increment(x=w447) -> (x+1=w446:i32)
        n184 = local read "Log File"() -> (w442:path)
        n185 = local read "Server copy Location"() -> (w439:path)
        n186 = Select(t=w446, s=w448, f=w447) -> (s? t:f=w445:i32)
        n187 = call "Write_File_Simple.vi"("append to file? (new file:F)"=TRUE, "character string"=w441, "file path"=w442) -> ("file path Out"=w440:path)  [unwired: 1 out]
        n188 = call "Updated_File_Copy.vi"("Target Path"=w439, "Source Path"=w440) -> ()  [unwired: 2 out]
      }
      frame 16 {
      }
      frame 17 {
        n189 = local read "Position Output XYZ"() -> (w488:dbl[])
        n190 = local read "Counters Reset?"() -> (w489:bool)
        n191 = Index Array(array=w488, index=2) -> (element=w494:dbl)
        n192 = Index Array(array=w488, index=0) -> (element=w496:dbl)
        n193 = Index Array(array=w488, index=1) -> (element=w495:dbl)
        n194 = Format Into String(format string="X= %.2f\tY= %.2f\tZ= %.2f" ("Format String"), w496, w495, w494) -> (resulting string=w497:string)  [unwired: 2 in, 1 out]
        n195 = case shown="\"Read traverse position\"" w481 {
          tunnel: w480 -> [w501 w503]
          tunnel: [w501 w502] -> w479
          frame "Move traverse", Default {
          }
          frame "Read traverse position" {
            n196 = Increment(x=w503) -> (x+1=w502:i32)
          }
        }
        n197 = Select(t="\nThe traverse was probably powered down since the last move. Its position has now been retaught and now all should be well.", s=w489, f="") -> (s? t:f=w490:string)
        n198 = call "Write_out_serial_log.vi"("Header message"=w497) -> ()
        n199 = Concatenate Strings(w485, w490) -> (w482:string)
        n200 = Empty String/Path?(string/path=w482) -> (empty?=w484:bool)
        n201 = Not(x=w484) -> (.not. x?=w483:bool)
      }
      frame 18 {
        # "Add demanded position"
        n202 = case shown="\"Work in Model Coordinates\"" w505 {
          tunnel: w508 -> [_ w523]
          tunnel: w507 -> [w518 w522]
          tunnel: [w518 w520] -> w506
          tunnel: [" (Tunnel Coordinates)" " (Model Coordinates)"] -> w504
          frame "Work in Tunnel Coordinates" {
          }
          frame "Work in Model Coordinates" {
            n203 = call "Coordinate_rotation.vi"("Model       Roll      Pitch       Yaw (deg)"=w523, "Input Position"=w522, "Mode"=T4."To User Coordinates") -> ("Output Position"=w520:dbl[])  [unwired: 2 in, 1 out]
          }
        }
        n204 = for {
          tunnel: w513 -> [w531] mode=indexing
          shift-right: [w526] -> w510
          shift-left: "\nDem Pos " -> [w529]
          tunnel: w506 -> [w524] mode=indexing
          n205 = Unbundle By Name(w531) -> ("Channel Properties.Channel Name"=w530:string)
          n206 = call "Split_Ch_name.vi"("Ch name"=w530) -> ("Low level"=w528:string)  [unwired: 2 out]
          n207 = Format Into String(format string="%s=%.1f, " ("Format String"), w528, w524) -> (resulting string=w525:string)  [unwired: 2 in, 1 out]
          n208 = Concatenate Strings(w529, w525) -> (w526:string)
        }
        n209 = Concatenate Strings(w511, w510, w504) -> (w509:string)
      }
      frame 19 {
        # "Add Achieved Position"
        n210 = local read "Position Output XYZ"() -> (w532:dbl[])
        n211 = case shown="\"Work in Model Coordinates\"" w533 {
          tunnel: w535 -> [_ w549]
          tunnel: [w546 w548] -> w534
          tunnel: w532 -> [w546 w547]
          frame "Work in Tunnel Coordinates" {
          }
          frame "Work in Model Coordinates" {
            n212 = call "Coordinate_rotation.vi"("Model       Roll      Pitch       Yaw (deg)"=w549, "Input Position"=w547, "Mode"=T4."To User Coordinates") -> ("Output Position"=w548:dbl[])  [unwired: 2 in, 1 out]
          }
        }
        n213 = for {
          tunnel: w542 -> [w561] mode=indexing
          shift-right: [w556] -> w539
          shift-left: "\nAchieved Pos " -> [w559]
          tunnel: w534 -> [w554] mode=indexing
          n214 = Unbundle By Name(w561) -> ("Channel Properties.Channel Name"=w560:string)
          n215 = call "Split_Ch_name.vi"("Ch name"=w560) -> ("Low level"=w558:string)  [unwired: 2 out]
          n216 = Format Into String(format string="%s=%.1f, " ("Format String"), w558, w554) -> (resulting string=w555:string)  [unwired: 2 in, 1 out]
          n217 = Concatenate Strings(w559, w555) -> (w556:string)
        }
        n218 = case shown="\"Move traverse\"" w537 {
          tunnel: ["When requesting a move." "When reading position." "When teaching position."] -> w536
          frame "Move traverse" {
          }
          frame "Read traverse position" {
          }
          frame "Teach Position" {
          }
        }
        n219 = Concatenate Strings(w540, w539, w536) -> (w538:string)
      }
    }
  }
  "Error String" <- w7
